vi "get data interface information.vi"(11 "fixed channel runtime in":refnum<class "control module runtime.lvclass">) -> (2 "data type defs":T1, 3 "fixed channel runtime out":refnum<class "control module runtime.lvclass">)   [LabVIEW 2013, in "control module runtime.lvclass"]
uses:
  control module runtime.lvclass
  data cluster type definition.ctl
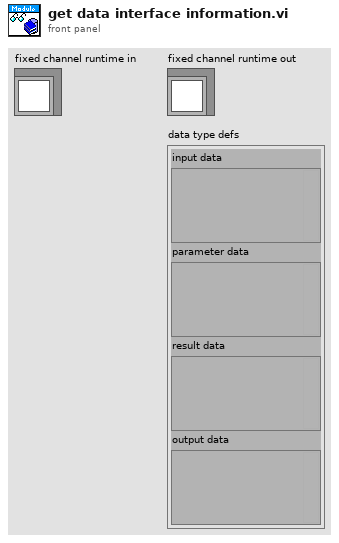
[diagram p1: front panel]
types:
  T1 = typedef "control module runtime.lvclass/data cluster type definition.ctl" = cluster{"input data":variant, "parameter data":variant, "result data":variant, "output data":variant}
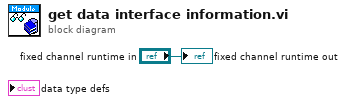
[diagram p0: block diagram]
diagram:
  "fixed channel runtime out" <- "fixed channel runtime in"
